vi "pkyk.vi"(8 "error in (no error)":errorcluster, 11 "New PKYK":T2) -> (0 "error out":errorcluster, 2 "MC No?":i32, 3 "PKYK":picture)   [LabVIEW 2020]
uses:
  Controls/PKYK_qData.ctl
  Controls/Poka_Status.ctl
  Controls/PKYK_Barcode_Status.ctl
  Controls/PKYK_Status.ctl
  Controls/Msg_Type.ctl
  MS SQL/MS_Global.vi
panel:
  out "Column":i16
  in  "Status":T1
  # "Required\nResult"
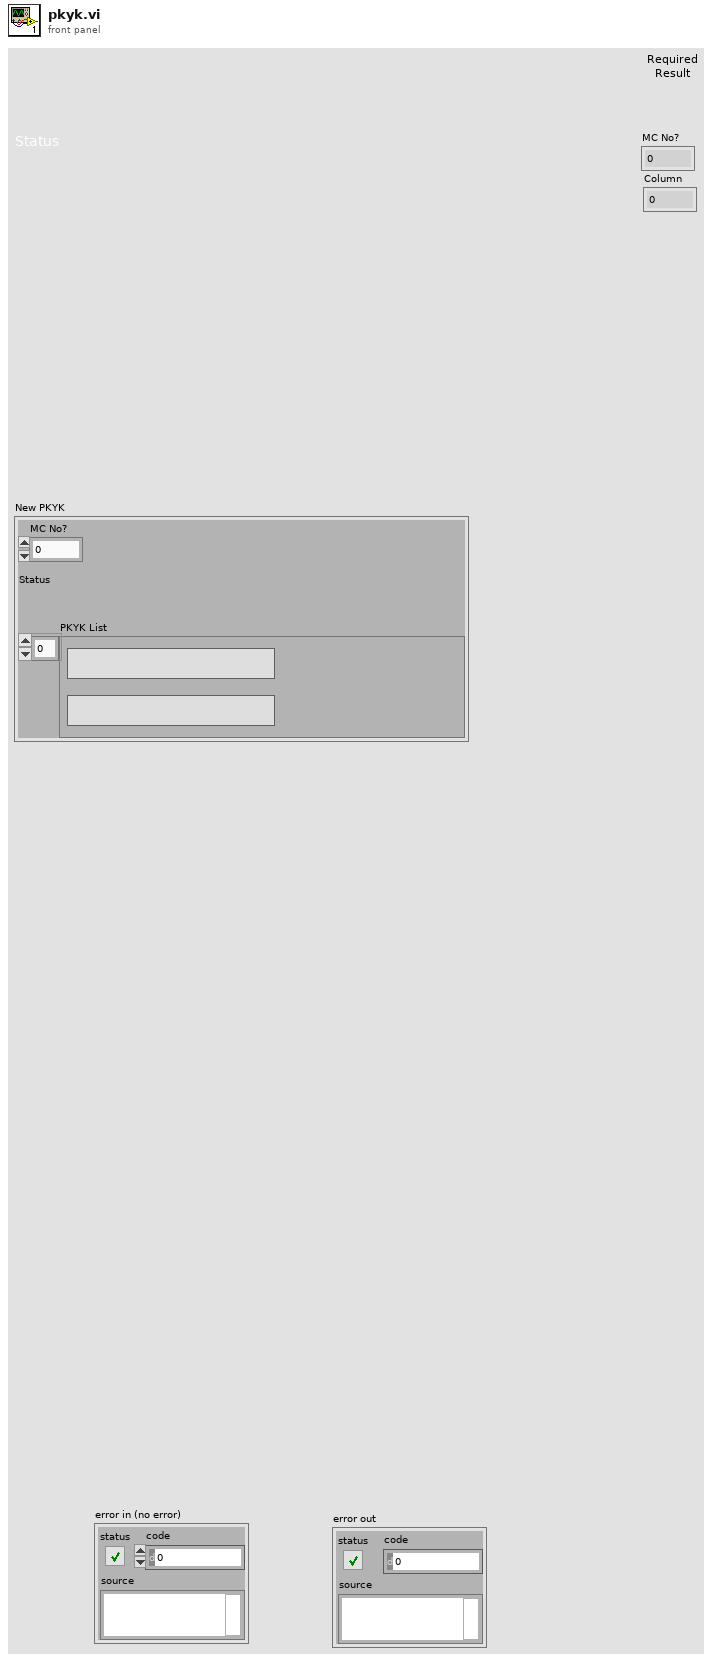
[diagram p1: front panel]
types:
  T1 = typedef "Poka_Status.ctl" = u16
  T2 = typedef "PKYK_qData.ctl" = cluster{"MC No?":i32, "Status":T1, "PKYK List":T3[]}
  T3 = typedef "PKYK_Barcode_Status.ctl" = cluster{"RFID Written Last":string, "Result":T4, "Exp. Result":T4}
  T4 = typedef "PKYK_Status.ctl" = u16
  T5 = typedef "Msg_Type.ctl" = enum16{"Normal", "Pass", "Fail", "Fault", "User", "Bypass", "Fail Save"}
  T6 = cluster{"left":i16, "top":i16, "right":i16, "bottom":i16}
  T7 = cluster{"Font Name:":string, "Size":i16, "Strikeout?":bool, "Italic?":bool, "Underline?":bool, "Outline?":bool, "Shadow?":bool, "Bold?":bool}
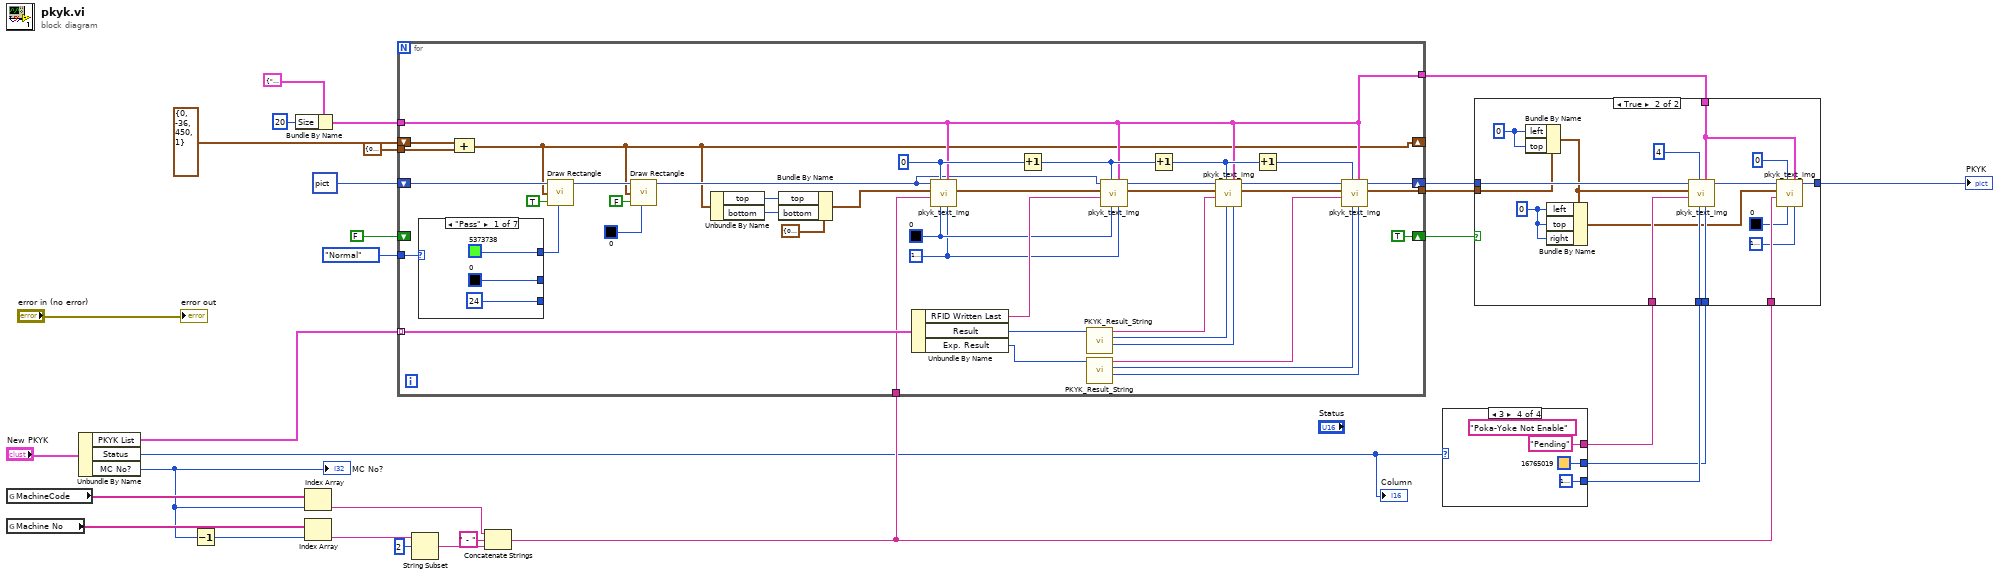
[diagram p0: block diagram]
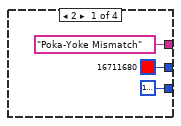
[diagram p3: hidden frame]
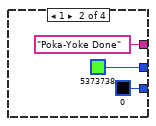
[diagram p4: hidden frame]
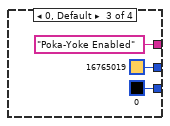
[diagram p5: hidden frame]
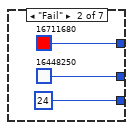
[diagram p6: hidden frame]
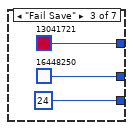
[diagram p7: hidden frame]
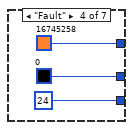
[diagram p8: hidden frame]
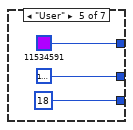
[diagram p9: hidden frame]
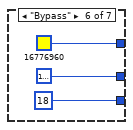
[diagram p10: hidden frame]
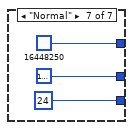
[diagram p11: hidden frame]
diagram:
  n1 = global read "MS_Global.vi" "MachineCode"() -> (w29:string[])
  n2 = global read "MS_Global.vi" "Machine No"() -> (w28:string[])
  n3 = Unbundle By Name("New PKYK") -> ("PKYK List"=w3:T3[], "Status"=w2:T1, "MC No?"=w1:i32)
  "MC No?" <- w1
  "Column" <- w2
  n4 = Decrement(x=w1) -> (x-1=w7:i32)
  n5 = Bundle By Name(cluster=T7 {"Font Name:"="Segoe UI Semibold", "Size"=18, "Strikeout?"=FALSE, "Italic?"=FALSE, "Underline?"=FALSE, "Outline?"=FALSE, "Shadow?"=FALSE, "Bold?"=FALSE} ("[user-specified font]"), "Size"=i16 20) -> (w22:T7)
  n6 = Index Array(array=w29, index=w1) -> (element=w20:string)
  n7 = Index Array(array=w28, index=w7) -> (element=w26:string)
  n8 = String Subset(string=w26, offset (0)=2) -> (substring=w19:string)  [unwired: 1 in]
  n9 = Concatenate Strings(w20, " - " ("string"), w19) -> (w8:string)
  n10 = for {
    tunnel: Msg_Type."Normal" ("Msg Type") -> [w67]
    tunnel: w22 -> [w34]
    tunnel: w8 -> [w60]
    tunnel: w3 -> [w65] mode=indexing
    shift-right: [w46] -> w12
    shift-left: picture data[5B] ("picture") -> [w64]
    shift-right: [w31] -> _
    shift-left: T6 {"left"=0, "top"=-36, "right"=450, "bottom"=1} ("output cluster") -> [w63]
    tunnel: T6 {"left"=0, "top"=36, "right"=0, "bottom"=36} ("output cluster") -> [w62]
    tunnel: [w35] -> w11
    tunnel: [w34] -> w10
    shift-right: [TRUE ("fill?(F)")] -> w4
    shift-left: FALSE ("fill?(F)") -> [_]
    w39 = i16 0 ("Column")
    w56 = u32 16777226 ("color(black)")
    w57 = u32 0 ("color(black)")
    n11 = case shown="\"Pass\"" w67 {
      tunnel: [u32 5373738 ("color(black)") u32 16711680 ("color(black)") u32 13041721 ("color(black)") u32 16745258 ("color(black)") u32 11534591 ("color(black)") u32 16776960 ("color(black)") u32 16448250 ("color(black)")] -> w66
      tunnel: [u32 0 ("color(black)") u32 16448250 ("color(black)") u32 16448250 ("color(black)") u32 0 ("color(black)") u32 16777226 ("color(black)") u32 16777222 ("color(black)") u32 16777222 ("color(black)")] -> _
      tunnel: [i16 24 ("Size") i16 24 ("Size") i16 24 ("Size") i16 24 ("Size") i16 18 ("Size") i16 18 ("Size") i16 24 ("Size")] -> _
      frame "Pass" {
      }
      frame "Fail" {
      }
      frame "Fail Save" {
      }
      frame "Fault" {
      }
      frame "User" {
      }
      frame "Bypass" {
      }
      frame "Normal" {
      }
    }
    n12 = Compound Arithmetic op=ADD(w63, w62) -> (w31:T6)
    n13 = call <vilib>:"Draw Rectangle.vi"("picture"=w64, "rect"=w31, "fill?(F)"=TRUE, "color(black)"=w66) -> ("new picture"=w69:picture)  [unwired: 5 in]
    n14 = call <vilib>:"Draw Rectangle.vi"("picture"=w69, "rect"=w31, "fill?(F)"=FALSE, "color(black)"=u32 0) -> ("new picture"=w33:picture)  [unwired: 5 in]
    n15 = Unbundle By Name(w31) -> ("top"=w42:i16, "bottom"=w41:i16)
    n16 = Bundle By Name(cluster=T6 {"left"=0, "top"=0, "right"=0, "bottom"=0} ("output cluster"), "top"=w42, "bottom"=w41) -> (w40:T6)
    n17 = Unbundle By Name(w65) -> ("RFID Written Last"=w58:string, "Result"=w61:T4, "Exp. Result"=w50:T4)
    n18 = call "pkyk_text_img.vi"("Fill Color"=w56, "[user-specified font]"=w34, "Text Color"=w57, "Column"=w39, "Text"=w60, "Orgin In"=w40, "new picture in"=w33) -> ("Orgin Out"=w59:T6)  [unwired: 3 in, 1 out]
    n19 = Increment(x=w39) -> (x+1=w38:i16)
    n20 = call "PKYK_Result_String.vi"("Result"=w61) -> ("color(black) 2"=w52:u32, "color(black)"=w53:u32, "RFID Written Last"=w45:string)  [unwired: 8 in]
    n21 = call "PKYK_Result_String.vi"("Result"=w50) -> ("color(black) 2"=w48:u32, "color(black)"=w49:u32, "RFID Written Last"=w44:string)  [unwired: 8 in]
    n22 = call "pkyk_text_img.vi"("Fill Color"=w56, "[user-specified font]"=w34, "Text Color"=w57, "Column"=w38, "Text"=w58, "Orgin In"=w59, "new picture in"=w33) -> ("Orgin Out"=w54:T6, "new picture out"=w55:picture)  [unwired: 3 in]
    n23 = Increment(x=w38) -> (x+1=w37:i16)
    n24 = call "pkyk_text_img.vi"("Fill Color"=w52, "[user-specified font]"=w34, "Text Color"=w53, "Column"=w37, "Text"=w45, "Orgin In"=w54, "new picture in"=w55) -> ("Orgin Out"=w51:T6, "new picture out"=w47:picture)  [unwired: 3 in]
    n25 = Increment(x=w37) -> (x+1=w36:i16)
    n26 = call "pkyk_text_img.vi"("Fill Color"=w48, "[user-specified font]"=w34, "Text Color"=w49, "Column"=w36, "Text"=w44, "Orgin In"=w51, "new picture in"=w47) -> ("Orgin Out"=w35:T6, "new picture out"=w46:picture)  [unwired: 3 in]
  }
  n27 = case shown="3" w2 {
    tunnel: ["Poka-Yoke Mismatch" ("Text") "Poka-Yoke Done" ("Text") "Poka-Yoke Enabled" ("Text") "Pending" ("Text")] -> w15
    tunnel: [u32 16777226 ("color(black)") u32 0 ("color(black)") u32 0 ("color(black)") u32 16777222 ("color(black)")] -> w14
    tunnel: [u32 16711680 ("color(black)") u32 5373738 ("color(black)") u32 16765019 ("color(black)") u32 16765019 ("color(black)")] -> w13
    frame 2 {
    }
    frame 1 {
    }
    frame 0, Default {
    }
    frame 3 {
      (unwired) "Poka-Yoke Not Enable" ("Text")
    }
  }
  n28 = case shown="True" w4 {
    tunnel: w15 -> [_ w122]
    tunnel: w14 -> [_ w121]
    tunnel: w13 -> [_ w120]
    tunnel: w12 -> [w105 w118]
    tunnel: w11 -> [_ w117]
    tunnel: w10 -> [_ w114]
    tunnel: [w105 w109] -> w9
    tunnel: w8 -> [_ w108]
    frame False {
    }
    frame True {
      w112 = i16 0 ("left")
      w116 = i16 0 ("left")
      n29 = Bundle By Name(cluster=w117, "left"=w116, "top"=w116) -> (w113:T6)
      n30 = Bundle By Name(cluster=w113, "left"=w112, "top"=w112, "right"=w112) -> (w111:T6)
      n31 = call "pkyk_text_img.vi"("Fill Color"=w120, "[user-specified font]"=w114, "Text Color"=w121, "Column"=i16 4, "Text"=w122, "Orgin In"=w113, "new picture in"=w118) -> ("new picture out"=w110:picture)  [unwired: 3 in, 1 out]
      n32 = call "pkyk_text_img.vi"("Fill Color"=u32 16777226 ("color(black)"), "[user-specified font]"=w114, "Text Color"=u32 0 ("color(black)"), "Column"=i16 0, "Text"=w108, "Orgin In"=w111, "new picture in"=w110) -> ("new picture out"=w109:picture)  [unwired: 3 in, 1 out]
    }
  }
  "PKYK" <- w9
  "error out" <- "error in (no error)"
